vi "close.vi"(6 "error in":errorcluster, 9 "Device Handle":u64) -> (0 "error out":errorcluster)   [LabVIEW 2018, in "Laser.lvlib"]
uses:
  Laser.lvlib
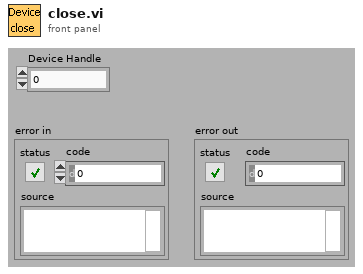
[diagram p1: front panel]
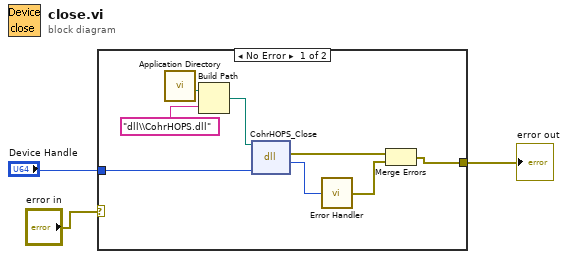
[diagram p0: block diagram]
diagram:
  n1 = case shown="No Error" "error in" {
    selector: "error in" -> [_ w12]
    tunnel: "Device Handle" -> [w11 _]
    tunnel: [w7 w12] -> w2
    frame No Error {
      n2 = call <vilib>:"Application Directory.vi"() -> ("Application Directory"=w6:path)
      n3 = Build Path(base path=w6, name or relative path="dll\\CohrHOPS.dll") -> (appended path=w4:path)
      n4 = dll-call lib="?" fn="CohrHOPS_Close"(path in=w4, "arg1"=w11) -> (error out=w8:errorcluster, "return type"=w10:i32)  [unwired: 3 in, 1 out]
      n5 = call "Error Handler.vi"("Return Value"=w10) -> ("error out"=w9:errorcluster)
      n6 = Merge Errors(w8, w9) -> (w7:errorcluster)
    }
    frame Error {
    }
  }
  "error out" <- w2
